vi "Query Instruments.vi"(8 "error in":errorcluster, 11 "Launcher in":refnum<class "Launcher.lvclass">) -> (0 "error out":errorcluster, 3 "Launcher out":refnum<class "Launcher.lvclass">)   [LabVIEW 2019, in "Launcher.lvlib" / "Launcher.lvclass"]
uses:
  Library/Launcher.lvclass
  Library/Launcher.lvclass/Launcher.ctl
  builds/Base Software/Base Software.lvlibp/Base Software Messages/Query Instruments Msg/Query Instruments Msg.lvclass
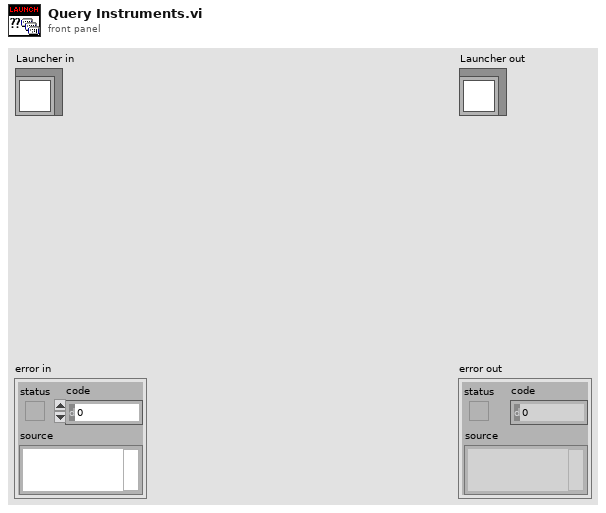
[diagram p1: front panel]
types:
  T1 = cluster{"Identifier":string, "Queue":refnum<class "Message Enqueuer.lvclass">}[]
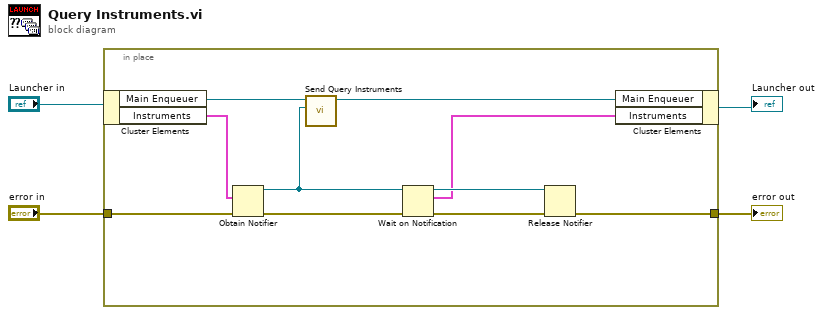
[diagram p0: block diagram]
diagram:
  n1 = in-place {
    in-place-border: "error in" -> [w10]
    in-place-border: [w8] -> w1
    n2 = in-place-cluster #1("Launcher in") -> ("Main Enqueuer"=w7:refnum<class "Message Enqueuer.lvclass">, "Instruments"=w11:T1)
    n3 = Obtain Notifier(notification data type=w11, error in (no error)=w10) -> (notifier out=w5:refnum<notifier>, error out=w13:errorcluster)  [unwired: 2 in, 1 out]
    n4 = call "Send Query Instruments.vi"("Instrument Notifier"=w5, "Message Enqueuer"=w7) -> ("Message Enqueuer out"=w6:refnum<class "Message Enqueuer.lvclass">)  [unwired: 8 in, 1 out]
    n5 = Wait on Notification(notifier=w5, error in (no error)=w13) -> (notifier out=w14:refnum<notifier>, notification=w9:T1, error out=w12:errorcluster)  [unwired: 2 in, 1 out]
    n6 = Release Notifier(notifier=w14, error in (no error)=w12) -> (error out=w8:errorcluster)  [unwired: 1 in, 2 out]
    n7 = in-place-cluster #1("Main Enqueuer"=w6, "Instruments"=w9) -> (→"Launcher out":refnum<class "Launcher.lvclass">)
  }
  "error out" <- w1
